vi "niRFUtil RFHS Channelizer RegisterFilter CSG_BlockSize.vi"(0 "Filter Spec":T2 {"Spec"."Flags" items=["None"=0, "Force Fractional"=1, "Use Multistage"=2, "Use Pretrigger Data "=256, "Frequency Shift Only"=4]; "Spec"."fs" format="%#_8p"; "Spec"."fc" format="%#_6p"; "Spec"."stopBW" format="%#_6p"; "Spec"."passBW" format="%#_6p"}, 5 "fs":dbl=1.0, 11 "error in (no error)":errorcluster) -> (4 "Filter Info":T1, 15 "error out":errorcluster)   [LabVIEW 2015, in "niRFUtil.lvlib"]
uses:
  niRFUtil.lvlib
  Includes/niRFUtil RFHS Channelizer FilterSpecification.ctl
  Includes/niRFUtil RFHS Channelizer ChannelSpecificationBase.ctl
  Includes/niRFUtil RFHS Channelizer ChannelFlags.ctl
  Includes/niRFUtil RFHS Filter Info.ctl
  niRFUtil RFHS Channelizer ChannelizerErrorToText.vi
  Includes/niRFUtil RFHS Channelizer FilterRef.ctl
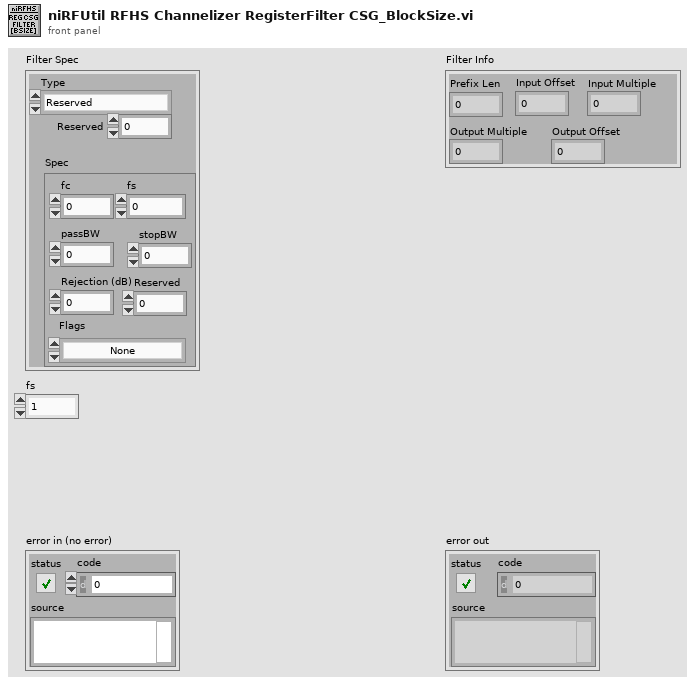
[diagram p1: front panel]
types:
  T1 = typedef "niRFUtil.lvlib/niRFUtil RFHS Filter Info.ctl" = cluster{"Prefix Len":i32, "Input Offset":i32, "Input Multiple":i32, "Output Multiple":dbl, "Output Offset":i32}
  T2 = typedef "niRFUtil.lvlib/niRFUtil RFHS Channelizer FilterSpecification.ctl" = cluster{"Type":enum32{"Reserved", "Rational", "Fine Tune", "Fractional", "Rational (user)", "Reserved 2", "Fractional (user)", "FFT Resampler"}, "Reserved":i32, "Spec":T3}
  T3 = typedef "niRFUtil.lvlib/niRFUtil RFHS Channelizer ChannelSpecificationBase.ctl" = cluster{"fc":dbl, "fs":dbl, "passBW":dbl, "stopBW":dbl, "Rejection (dB)":dbl, "Flags":T4, "Reserved":i32}
  T4 = typedef "niRFUtil.lvlib/niRFUtil RFHS Channelizer ChannelFlags.ctl" = u32
  T5 = typedef "niRFUtil.lvlib/niRFUtil RFHS Channelizer FilterRef.ctl" = cluster{"Ref":u64, "GUID":u64, "Upsample":i32, "Downsample":i32, "Size":i32, "Num Taps":i32}
  T6 = enum32{"Reserved", "Rational", "Fine Tune", "Fractional", "Rational (user)", "Reserved 2", "Fractional (user)", "FFT Resampler"}
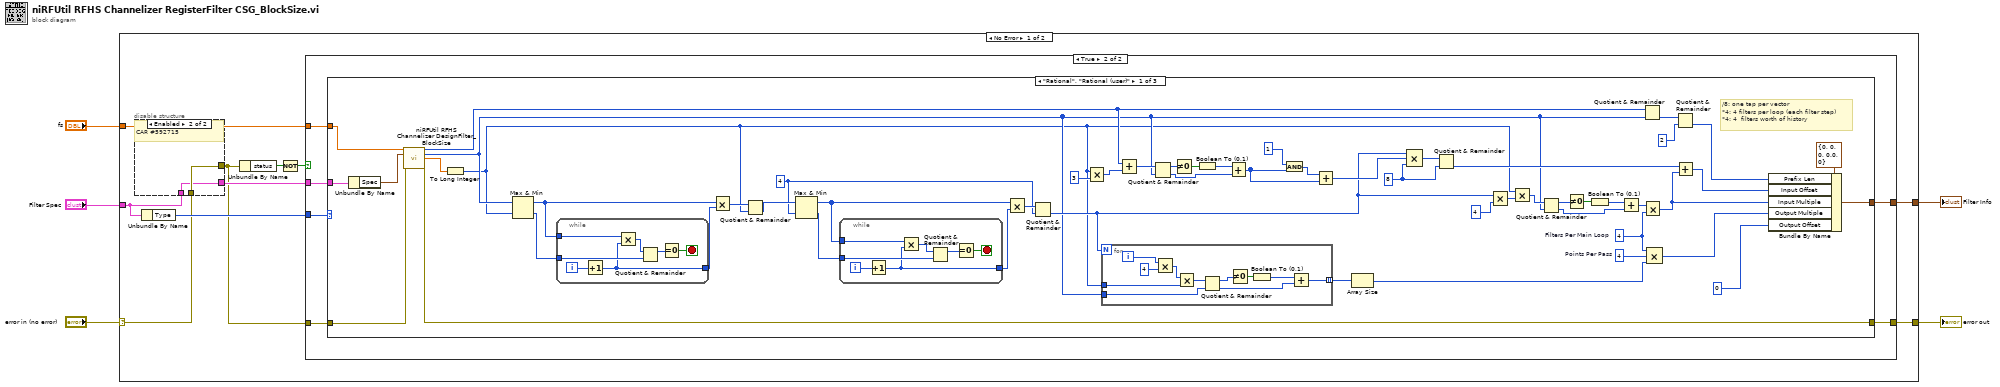
[diagram p0: block diagram]
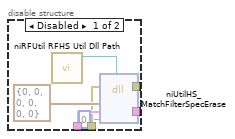
[diagram p2: hidden frame]
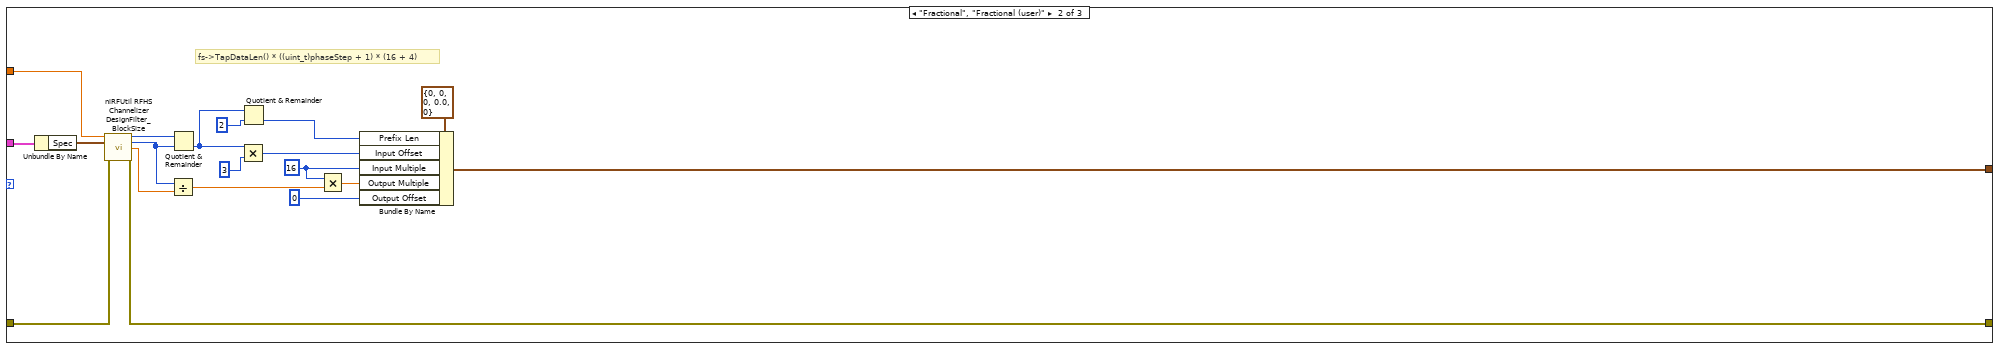
[diagram p4: hidden frame]
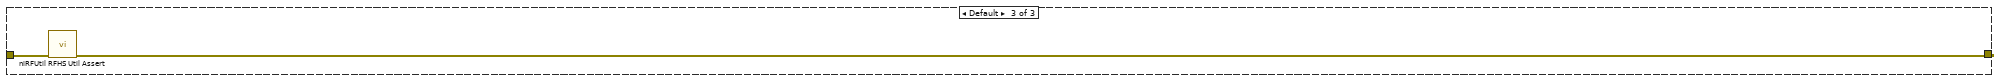
[diagram p5: hidden frame]
diagram:
  n1 = case shown="No Error" "error in (no error)" {
    selector: "error in (no error)" -> [w11 w133]
    tunnel: "Filter Spec" -> [w13 _]
    tunnel: "fs" -> [w14 _]
    tunnel: [w8 w133] -> w2
    tunnel: [w7 _] -> w1
    frame No Error {
      n2 = disable-structure shown="Enabled" {
        disable-tunnel: [w20 w23] -> w15
        disable-tunnel: w13 -> [w19 w23]
        disable-tunnel: w11 -> [w18 w24]
        disable-tunnel: [w17 w24] -> w6
        frame Disabled {
          n3 = call "niRFUtil RFHS Util Dll Path.vi"() -> ("Path"=w21:path)  [unwired: 7 in, 4 out]
          n4 = dll-call lib="?" fn="niUtilHS_MatchFilterSpecErase"(path in=w21, error in=w18, "lvRef"=T5 {"Ref"=0, "GUID"=0, "Upsample"=0, "Downsample"=0, "Size"=0, "Num Taps"=0} ("LVRef"), "filterSpec"=w19, "erase"=0) -> (error out=w17:errorcluster, "filterSpec"=w20:T2)  [unwired: 4 in, 1 out]
        }
        frame Enabled {
          # "CAR #592715"
        }
      }
      n5 = Unbundle By Name(w13) -> ("Type"=w12:T6)
      n6 = Unbundle By Name(w6) -> ("status"=w10:bool)
      n7 = Not(x=w10) -> (.not. x?=w9:bool)
      n8 = case shown="True" w9 {
        tunnel: w15 -> [_ w30]
        tunnel: w14 -> [_ w31]
        tunnel: w12 -> [_ w29]
        tunnel: w6 -> [w25 w28]
        tunnel: [w25 w27] -> w8
        tunnel: [_ w26] -> w7
        frame False {
        }
        frame True {
          n9 = case shown="\"Rational\", \"Rational (user)\"" w29 {
            tunnel: w31 -> [w67 w130 _]
            tunnel: w30 -> [w66 w129 _]
            tunnel: w28 -> [w65 w128 w132]
            tunnel: [w57 w126 w131] -> w27
            tunnel: [w55 w117 _] -> w26
            frame "Rational", "Rational (user)" {
              w47 = 4  # Points Per Pass
              w48 = 4  # Filters Per Main Loop
              w38 = 8 ("y")
              w81 = 4
              # "/8: one tap per vector\n*4: 4 filters per loop (each filter step)\n*4: 4  filters worth of history"
              n10 = Unbundle By Name(w66) -> ("Spec"=w62:T3)
              n11 = call "niRFUtil RFHS Channelizer DesignFilter_BlockSize.vi"("fs"=w67, "Channel Specification"=w62, "error in (no error)"=w65) -> ("Filter Taps"=w39:i32, "upsample"=w35:i32, "downsample"=w63:dbl, "error out"=w57:errorcluster)  [unwired: 9 in]
              n12 = To Long Integer(number=w63) -> (32bit integer=w34:i32)
              n13 = Max & Min(x=w35, y=w34) -> (max(x,y)=w44:i32, min(x,y)=w86:i32)
              n14 = while {
                tunnel: w86 -> [w111]
                tunnel: [w106] -> w43
                tunnel: w44 -> [w105]
                i -> [w108]
                stop <- w109 stop-if-true
                n15 = Increment(x=w108) -> (x+1=w106:i32)
                n16 = Multiply(x=w105, y=w106) -> (x*y=w107:i32)
                n17 = Quotient & Remainder(x=w107, y=w111) -> (x-y*floor(x/y)=w110:i32)  [unwired: 1 out]
                n18 = Equal To 0?(x=w110) -> (x = 0?=w109:bool)
              }
              n19 = Multiply(x=w44, y=w43) -> (x*y=w85:i32)
              n20 = Quotient & Remainder(x=w85, y=w34) -> (floor(x/y)=w83:i32)  [unwired: 1 out]
              n21 = Max & Min(x=w83, y=w81) -> (max(x,y)=w41:i32, min(x,y)=w84:i32)
              n22 = while {
                tunnel: w84 -> [w104]
                tunnel: [w99] -> w42
                tunnel: w41 -> [w100]
                i -> [w101]
                stop <- w102 stop-if-true
                n23 = Increment(x=w101) -> (x+1=w99:i32)
                n24 = Multiply(x=w100, y=w99) -> (x*y=w98:i32)
                n25 = Quotient & Remainder(x=w98, y=w104) -> (x-y*floor(x/y)=w103:i32)  [unwired: 1 out]
                n26 = Equal To 0?(x=w103) -> (x = 0?=w102:bool)
              }
              n27 = Multiply(x=w41, y=w42) -> (x*y=w82:i32)
              n28 = Quotient & Remainder(x=w82, y=w81) -> (floor(x/y)=w36:i32)  [unwired: 1 out]
              n29 = Multiply(x=w34, y=3) -> (x*y=w40:i32)
              n30 = for {
                N: w36 -> [_]
                tunnel: w35 -> [w91]
                tunnel: w34 -> [w94]
                tunnel: [w87] -> w51 mode=indexing
                i -> [w97]
                n31 = Multiply(x=w97, y=4) -> (x*y=w95:i32)
                n32 = Multiply(x=w95, y=w94) -> (x*y=w93:i32)
                n33 = Quotient & Remainder(x=w93, y=w91) -> (x-y*floor(x/y)=w92:i32, floor(x/y)=w88:i32)
                n34 = Not Equal To 0?(x=w92) -> (x != 0?=w90:bool)
                n35 = Boolean To (0,1)(Boolean=w90) -> (0, 1=w89:i16)
                n36 = Add(x=w89, y=w88) -> (x+y=w87:i32)
              }
              n37 = Add(x=w39, y=w40) -> (x+y=w58:i32)
              n38 = Quotient & Remainder(x=w58, y=w35) -> (x-y*floor(x/y)=w80:i32, floor(x/y)=w77:i32)
              n39 = Not Equal To 0?(x=w80) -> (x != 0?=w79:bool)
              n40 = Boolean To (0,1)(Boolean=w79) -> (0, 1=w78:i16)
              n41 = Add(x=w78, y=w77) -> (x+y=w75:i32)
              n42 = And(x=1, y=w75) -> (x .and. y?=w74:i32)
              n43 = Add(x=w74, y=w75) -> (x+y=w61:i32)
              n44 = Array Size(array=w51) -> (size(s)=w46:i32)
              n45 = Compound Arithmetic op=MULTIPLY(w36, w61, w38) -> (w60:i32)
              n46 = Quotient & Remainder(x=w60, y=w38) -> (floor(x/y)=w64:i32)  [unwired: 1 out]
              n47 = Multiply(x=w36, y=4) -> (x*y=w37:i32)
              n48 = Multiply(x=w34, y=w37) -> (x*y=w72:i32)
              n49 = Quotient & Remainder(x=w72, y=w35) -> (x-y*floor(x/y)=w73:i32, floor(x/y)=w68:i32)
              n50 = Not Equal To 0?(x=w73) -> (x != 0?=w70:bool)
              n51 = Boolean To (0,1)(Boolean=w70) -> (0, 1=w69:i16)
              n52 = Add(x=w69, y=w68) -> (x+y=w50:i32)
              n53 = Quotient & Remainder(x=w39, y=w35) -> (floor(x/y)=w53:i32)  [unwired: 1 out]
              n54 = Multiply(x=w50, y=w48) -> (x*y=w33:i32)
              n55 = Compound Arithmetic op=MULTIPLY(w48, w47, w46) -> (w45:i32)
              n56 = Quotient & Remainder(x=w53, y=2) -> (floor(x/y)=w54:i32)  [unwired: 1 out]
              n57 = Add(x=w64, y=w33) -> (x+y=w49:i32)
              n58 = Bundle By Name(cluster=T1 {"Prefix Len"=0, "Input Offset"=0, "Input Multiple"=0, "Output Multiple"=0.0, "Output Offset"=0} ("Filter Info 2"), "Prefix Len"=w54, "Input Offset"=w49, "Input Multiple"=w33, "Output Multiple"=w45, "Output Offset"=0) -> (w55:T1)
            }
            frame "Fractional", "Fractional (user)" {
              w115 = 16 ("Input Multiple")
              # "fs->TapDataLen() * ((uint_t)phaseStep + 1) * (16 + 4)"
              n59 = Unbundle By Name(w129) -> ("Spec"=w127:T3)
              n60 = call "niRFUtil RFHS Channelizer DesignFilter_BlockSize.vi"("fs"=w130, "Channel Specification"=w127, "error in (no error)"=w128) -> ("Filter Taps"=w123:i32, "upsample"=w116:i32, "downsample"=w112:dbl, "error out"=w126:errorcluster)  [unwired: 9 in]
              n61 = Divide(x=w116, y=w112) -> (x/y=w114:dbl)
              n62 = Quotient & Remainder(x=w123, y=w116) -> (floor(x/y)=w120:i32)  [unwired: 1 out]
              n63 = Multiply(x=w120, y=3) -> (x*y=w121:i32)
              n64 = Quotient & Remainder(x=w120, y=2) -> (floor(x/y)=w119:i32)  [unwired: 1 out]
              n65 = Multiply(x=w115, y=w114) -> (x*y=w113:dbl)
              n66 = Bundle By Name(cluster=T1 {"Prefix Len"=0, "Input Offset"=0, "Input Multiple"=0, "Output Multiple"=0.0, "Output Offset"=0} ("Filter Info 2"), "Prefix Len"=w119, "Input Offset"=w121, "Input Multiple"=w115, "Output Multiple"=w113, "Output Offset"=0) -> (w117:T1)
            }
            frame Default {
              n67 = call "niRFUtil RFHS Util Assert.vi"("error constant"=w132) -> ("error constant 3"=w131:errorcluster)  [unwired: 14 in]
            }
          }
        }
      }
    }
    frame Error {
    }
  }
  "error out" <- w2
  "Filter Info" <- w1
